vi "getClassHierarchyFromClassName.vi"(8 "error in (no error)":errorcluster, 11 "className":string) -> (0 "error out":errorcluster, 3 "hierarchy":string[](array[string]))   [LabVIEW 2023, in "TLC_Scripto.lvlib"]
uses:
  TLC_Scripto.lvlib
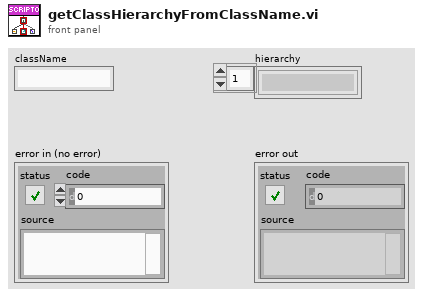
[diagram p1: front panel]
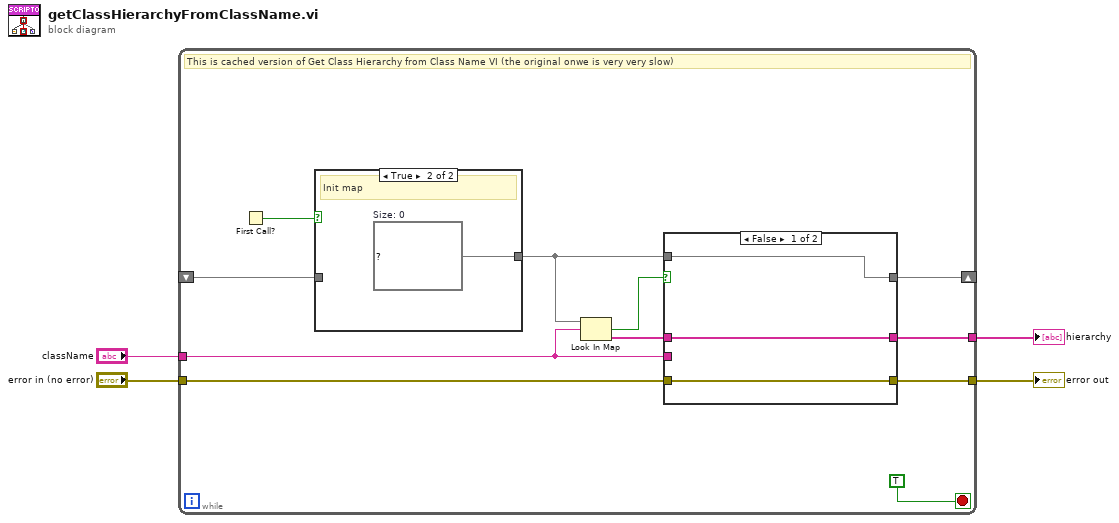
[diagram p0: block diagram]
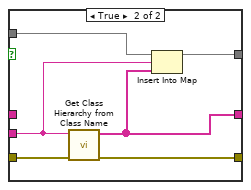
[diagram p3: hidden frame]
diagram:
  n1 = while {
    tunnel: "className" -> [w13]
    tunnel: "error in (no error)" -> [w15]
    tunnel: [w10] -> w2
    shift-right: [w9] -> _
    shift-left: _ -> [w6]
    tunnel: [w5] -> w1
    stop <- TRUE stop-if-true
    # "This is cached version of Get Class Hierarchy from Class Name VI (the original onwe is very very slow)"
    n2 = First Call?() -> (First Call?: T/F=w8:bool)
    n3 = case shown="True" w8 {
      tunnel: [w16 w17] -> w7
      tunnel: w6 -> [w16 _]
      frame False {
      }
      frame True {
        w17 = map{string, string[]} {}  # Size: 0
        # "Init map"
      }
    }
    n4 = Look In Map(map=w7, key=w13) -> (key not found?=w12:bool, value=w11:string[])  [unwired: 1 in]
    n5 = case shown="False" w12 {
      tunnel: w13 -> [_ w24]
      tunnel: w15 -> [w18 w26]
      tunnel: w11 -> [w20 _]
      tunnel: [w20 w22] -> w10
      tunnel: w7 -> [w19 w25]
      tunnel: [w19 w23] -> w9
      tunnel: [w18 w21] -> w5
      frame False {
      }
      frame True {
        n6 = call <vilib>:"Get Class Hierarchy from Class Name.vi"("error in (no error)"=w26, "Class Name"=w24) -> ("error out"=w21:errorcluster, "Class Hierarchy"=w22:string[])  [unwired: 8 in]
        n7 = Insert Into Map(map in=w25, key=w24, value=w22) -> (map out=w23:map{string, string[]})  [unwired: 2 out]
      }
    }
  }
  "hierarchy" <- w2
  "error out" <- w1
